vi "Make PWM JSON.vi"(9 "Force":bool, 10 "PWM prev":T1, 11 "PWM new":T1) -> (3 "delta JSON":string)   [LabVIEW 2019]
uses:
  PWM data proto.ctl
  PWM proto.ctl
panel:
  out "Complete JSON":string
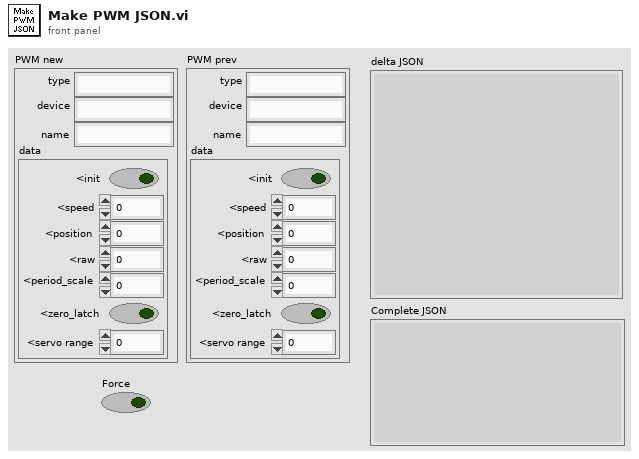
[diagram p1: front panel]
types:
  T1 = typedef "PWM proto.ctl" = cluster{"type":string, "device":string, "name":string, "data":T2}
  T2 = typedef "PWM data proto.ctl" = cluster{"<init":bool, "<speed":dbl, "<position":dbl, "<raw":dbl, "<period_scale":dbl, "<zero_latch":bool, "<servo range":dbl}
  T3 = cluster{"type":bool, "device":bool, "name":bool, "data":cluster{"<init":bool, "<speed":bool, "<position":bool, "<raw":bool, "<period_scale":bool, "<zero_latch":bool, "<servo range":bool}}
  T4 = cluster{"<init":bool, "<speed":bool, "<position":bool, "<raw":bool, "<period_scale":bool, "<zero_latch":bool, "<servo range":bool}
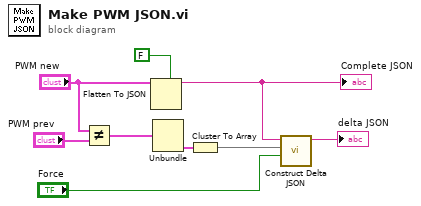
[diagram p0: block diagram]
diagram:
  n1 = Not Equal?(x="PWM new", y="PWM prev") -> (x != y?=w1:T3)
  n2 = Flatten To JSON(enable LabVIEW extensions? (T)=FALSE, anything="PWM new") -> (JSON string=w8:string)  [unwired: 1 in, 1 out]
  "Complete JSON" <- w8
  n3 = Unbundle(w1) -> ("data"=w4:T4)  [unwired: 3 out]
  n4 = Cluster To Array(cluster=w4) -> (array=w2:bool[])
  n5 = call "Construct Delta JSON.vi"("Force"="Force", "Checked Items"=w2, "JSON string"=w8) -> ("Delta JSON"=→"delta JSON":string)  [unwired: 8 in]
